vi "Project Names.vi"(8 "Error In":errorcluster, 11 "App In":refnum<vi>) -> (0 "Error Out":errorcluster, 2 "Project Names":string[](array[string]), 3 "App Out":refnum<vi>)   [LabVIEW 2017, in "Bookmark Manager.lvlib"]
uses:
  Bookmark Manager.lvlib
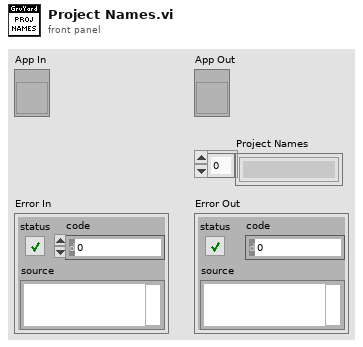
[diagram p1: front panel]
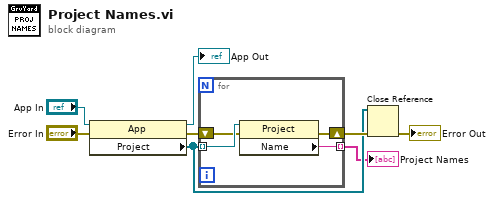
[diagram p0: block diagram]
diagram:
  n1 = property class="App"(reference="App In", error in="Error In") -> (reference out=→"App Out":refnum<vi>, error out=w7:errorcluster, "Project"=w5:refnum<vi>[])
  n2 = for {
    shift-right: [w10] -> w6
    shift-left: w7 -> [w11]
    tunnel: w5 -> [w12] mode=indexing
    tunnel: [w9] -> w1 mode=indexing
    n3 = property class="Project"(reference=w12, error in=w11) -> (error out=w10:errorcluster, "Name"=w9:string)  [unwired: 1 out]
  }
  "Project Names" <- w1
  n4 = Close Reference(reference=w5, error in (no error)=w6) -> (error out=→"Error Out":errorcluster)
